vi "Python_Init.vi"(1 "code in":path, 2 "error in (no error)":errorcluster) -> (3 "Refnum out":refnum<k35>, 4 "code":path, 6 "error out":errorcluster)   [LabVIEW 2025]
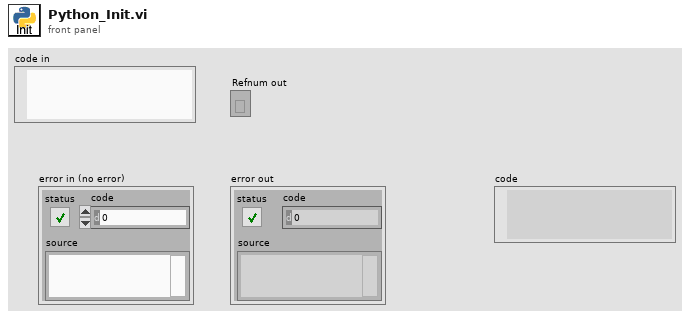
[diagram p1: front panel]
types:
  T1 = cluster{"Python version":string, "Python path":string}
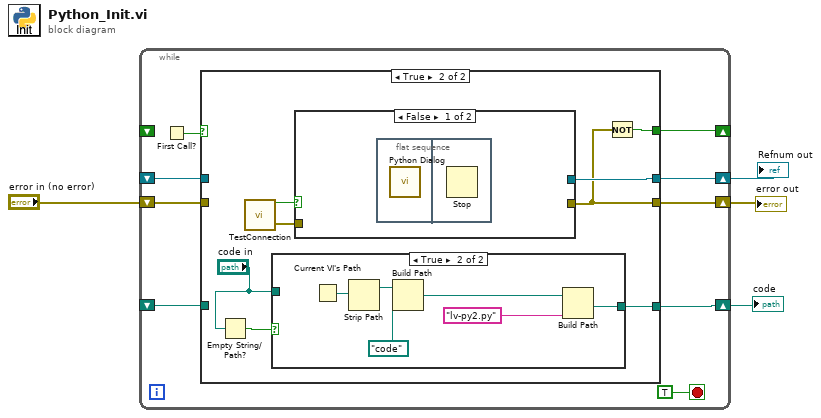
[diagram p0: block diagram]
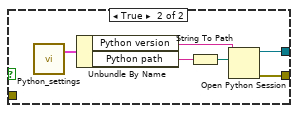
[diagram p4: hidden frame]
diagram:
  n1 = while {
    shift-right: [w13] -> w4
    shift-left: "error in (no error)" -> [w11]
    shift-right: [w10] -> _
    shift-left: _ -> [_]
    shift-right: [w12] -> w3
    shift-left: _ -> [w9]
    shift-right: [w6] -> w1
    shift-left: _ -> [w5]
    stop <- TRUE stop-if-true
    n2 = First Call?() -> (First Call?: T/F=w7:bool)
    n3 = case shown="True" w7 {
      selector: w7 -> [w17 _]
      tunnel: [w15 w23] -> w13
      tunnel: [w16 w24] -> w12
      tunnel: w11 -> [w15 _]
      tunnel: [w17 w25] -> w10
      tunnel: w9 -> [w16 _]
      tunnel: [w14 w19] -> w6
      tunnel: w5 -> [w14 _]
      frame False {
      }
      frame True {
        n4 = Empty String/Path?(string/path="code in") -> (empty?=w21:bool)
        n5 = call "TestConnection.vi"() -> ("error out"=w18:errorcluster, "success?"=w22:bool)  [unwired: 2 in]
        n6 = case shown="True" w21 {
          tunnel: [w26 w28] -> w19
          tunnel: "code in" -> [w26 _]
          frame False {
          }
          frame True {
            n7 = Current VI's Path() -> (path=w29:path)
            n8 = Strip Path(path=w29) -> (stripped path=w30:path)  [unwired: 1 out]
            n9 = Build Path(base path=w30, name or relative path=path "code") -> (appended path=w27:path)
            n10 = Build Path(base path=w27, name or relative path="lv-py2.py") -> (appended path=w28:path)
          }
        }
        n11 = case shown="False" w22 {
          tunnel: [_ w38] -> w24
          tunnel: [_ w37] -> w23
          tunnel: w18 -> [_ _]
          frame False {
            n12 = flat-sequence {
              frame #0 {
                n13 = call "Python Dialog.vi"() -> ()  [unwired: 12 in]
              }
              frame #1 {
                n14 = Stop() -> ()  [unwired: 1 in]
              }
            }
          }
          frame True {
            n15 = call "Python_settings.vi"() -> ("settings read"=w35:T1)  [unwired: 5 in]
            n16 = Unbundle By Name(w35) -> ("Python version"=w33:string, "Python path"=w36:string)
            n17 = String To Path(string=w36) -> (path=w34:path)
            n18 = Open Python Session(python version=w33, python path=w34) -> (session out=w38:refnum<k35>, error out=w37:errorcluster)  [unwired: 1 in]
          }
        }
        n19 = Not(x=w23) -> (.not. x?=w25:bool)
      }
    }
  }
  "error out" <- w4
  "Refnum out" <- w3
  "code" <- w1
